vi "readPress03.vi"() -> ()   [LabVIEW 2011]
uses:
  Growth Sequences/Control 1.ctl
  <vilib>/Instr/_visa.llb/VISA Configure Serial Port (Instr).vi
panel:
  out "return count":u32
  in  "delay before read (ms)":u32=500
  in  "y":i32=1000
  in  "VISA resource name":T1="COM1"
  out "read buffer":string
  out "P (Torr)":dbl
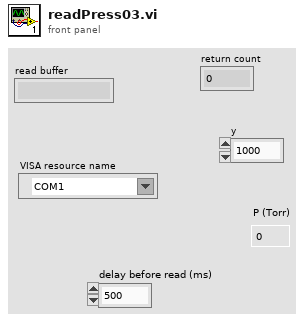
[diagram p1: front panel]
types:
  T1 = typedef "Control 1.ctl" = refnum<visa-resource-name>
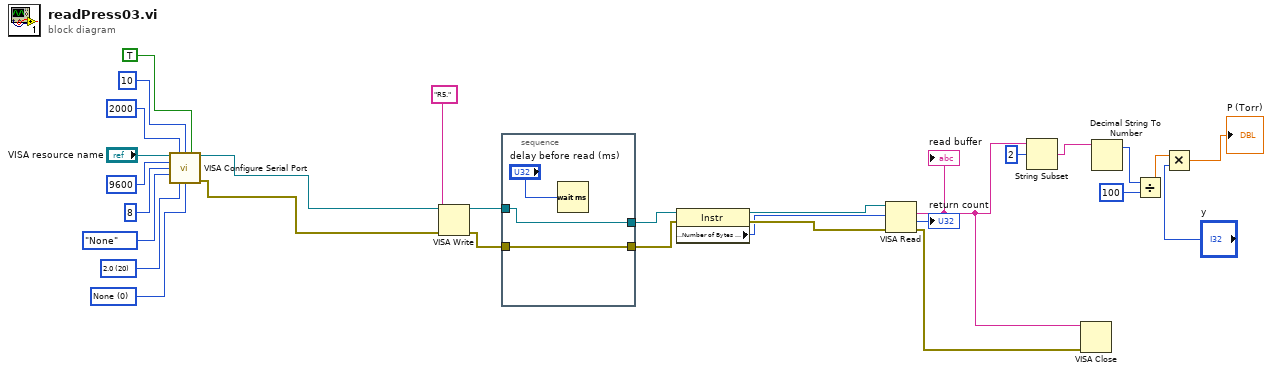
[diagram p0: block diagram]
diagram:
  w8 = u16 0 items=["None", "XON/XOFF", "RTS/CTS", "XON/XOFF & RTS/CTS", "DTR/DSR", "XON/XOFF & DTR/DSR"] ("flow control (0:none)")
  w9 = u16 20 items=["1.0"=10, "1.5"=15, "2.0"=20] ("stop bits (10: 1 bit)")
  n1 = call-poly "VISA Configure Serial Port"("VISA resource name"="VISA resource name", "timeout (10sec)"=u32 2000 ("General Settings:Timeout Value"), "termination char\n(0xA = '\\n' = LF)"=u8 10 ("termination char\n(0xA = '\\n' = LF)"), "Enable Termination\nChar (T)"=TRUE ("Enable Termination\nChar (T)"), "baud rate (9600)"=u32 9600, "data bits (8)"=u16 8, "parity (0:none)"=enum16{"None", "Odd", "Even", "Mark", "Space"}."None", "stop bits (10: 1 bit)"=w9, "flow control (0:none)"=w8) -> ("VISA resource name out"=w2:refnum<visa-resource-name>, "error out"=w1:errorcluster)  [unwired: 5 in]
  n2 = VISA Write(VISA resource name=w2, write buffer="R5.", error in (no error)=w1) -> (VISA resource name out=w21:refnum<visa-resource-name>, error out=w20:errorcluster)  [unwired: 1 out]
  n3 = stacked-sequence {
    tunnel: w20 -> [w32]
    tunnel: [w32] -> w18
    tunnel: [w30] -> w19
    tunnel: w21 -> [w30]
    frame #0 {
      n4 = Wait (ms)(milliseconds to wait="delay before read (ms)") -> ()  [unwired: 1 out]
    }
  }
  n5 = property class="Instr"(reference=w19, error in=w18) -> (reference out=w16:refnum<visa-resource-name>, error out=w17:errorcluster, "Serial Settings:Number of Bytes at Serial Port"=w15:u32)
  n6 = VISA Read(VISA resource name=w16, byte count=w15, error in (no error)=w17) -> (read buffer=w5:string, return count=→"return count":u32, error out=w4:errorcluster)  [unwired: 1 out]
  "read buffer" <- w5
  n7 = String Subset(string=w5, offset (0)=2) -> (substring=w29:string)  [unwired: 1 in]
  n8 = VISA Close(VISA resource name=w5, error in (no error)=w4) -> ()  [unwired: 1 out]
  n9 = Decimal String To Number(string=w29) -> (offset past number=w24:i32)  [unwired: 2 in, 1 out]
  n10 = Divide(x=w24, y=100) -> (x/y=w22:dbl)
  n11 = Multiply(x=w22, y="y") -> (x*y=→"P (Torr)":dbl)
